vi "Write to XML File.vi"   [LabVIEW 2020]
doc: "Writes a text string of XML data with accompanying header tags to a text file. Wire data to the <B>XML Input</B> input to determine the polymorphic instance to use or manually select the instance. All XML data must follow the standard LabVIEW XML schema."
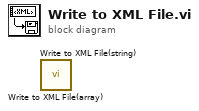
[diagram p0: block diagram]
diagram:
  n1 = call "Write to XML File(array).vi"() -> ()  [unwired: 9 in, 3 out]
  n2 = call "Write to XML File(string).vi"() -> ()  [unwired: 9 in, 3 out]
